vi "ELOG_OutputFormat_Set.vi"(8 "error in (no error)":errorcluster, 10 "Output Format":T1, 11 "OXY_SCPI Reseource In":refnum<visa-resource-name>) -> (0 "error out":errorcluster, 1 "communication_data":T2, 3 "OXY_SCPI Reseource Out":refnum<visa-resource-name>)   [LabVIEW 2018, in "OXYGEN.lvlib"]
doc: "Sets the requested output format."
uses:
  OXYGEN.lvlib
  TypeDefs/Cluster_RawCommData.ctl
  TypeDefs/Enum_ELOGOutputFomarts.ctl
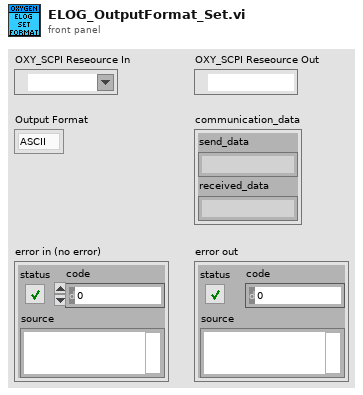
[diagram p1: front panel]
types:
  T1 = typedef "OXYGEN.lvlib/Enum_ELOGOutputFomarts.ctl" = enum16{"ASCII", "BIN_INTEL", "BIN_MOTOROLA"}
  T2 = typedef "OXYGEN.lvlib/Cluster_RawCommData.ctl" = cluster{"send_data":string, "received_data":string}
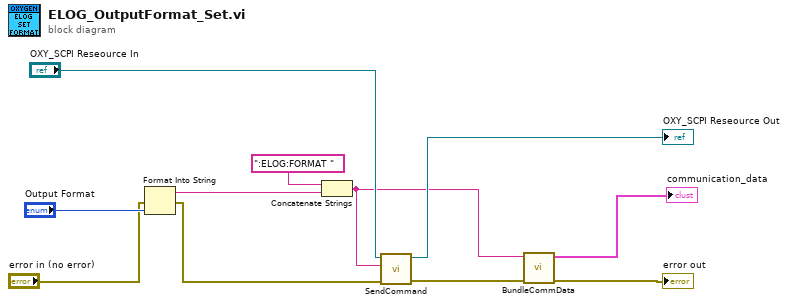
[diagram p0: block diagram]
diagram:
  n1 = Format Into String(error in="error in (no error)", "Output Format") -> (resulting string=w3:string, error out=w1:errorcluster)  [unwired: 2 in]
  n2 = Concatenate Strings(":ELOG:FORMAT " ("string"), w3) -> (w8:string)
  n3 = call "SendCommand.vi"("error in (no error)"=w1, "String to Send"=w8, "OXY_SCPI Reseource In"="OXY_SCPI Reseource In") -> ("error out"=w5:errorcluster, "OXY_SCPI Reseource Out"=→"OXY_SCPI Reseource Out":refnum<visa-resource-name>)  [unwired: 7 in]
  n4 = call "BundleCommData.vi"("error in (no error)"=w5, "send_data"=w8) -> ("error out"=→"error out":errorcluster, "communication_data"=→"communication_data":T2)  [unwired: 8 in]
